vi "Write Ch.vi"(8 "error in":errorcluster, 9 "Channel":i32, 10 "Producer Ch":T1, 11 "Cycler Cluster - 24 Channel.lvclass":refnum<class "Cycler Cluster - 24 Channel.lvclass">) -> (0 "error out":errorcluster, 3 "output cluster":refnum<class "Cycler Cluster - 24 Channel.lvclass">)   [LabVIEW 2023, in "Cycler Cluster - 24 Channel.lvclass"]
uses:
  Cycler Cluster - 24 Channel.lvclass
  Cycler Cluster - 24 Channel.lvclass/Cycler Cluster - 24 Channel.ctl
  f4d7046b-01d5-476e-969f-edff788d7dd0.vi
  09ba8855-a333-4b05-9fa0-f00f0d112976.vi
  f692a3ce-3a89-48d1-896d-de4404ed547f.vi
  300b3033-2680-412c-ab22-c723e8d8dc08.vi
  7cf0eb00-689e-4e52-8b4d-642b65507f98.vi
  b87ff49e-8005-4a7c-bf49-406770351efc.vi
  dc6f3a3c-9a41-4b47-836c-8d10a2dd6bc9.vi
  5b0f37a0-0270-4c49-ba01-7464d39b0c09.vi
  d2784768-1ffd-4bb1-aa68-cb021ec6bd11.vi
  d58bec58-6c3c-4b44-9526-a74563a41a00.vi
  6f99bfdc-e3a0-47bf-9a28-a7b183ece507.vi
  03bc517d-3567-4243-82ce-a9681bd71644.vi
  cfb328b4-c11e-4fec-8c64-e5bccd80eed6.vi
  f724775c-be9e-4d2c-be3a-0a88198af531.vi
  bbda8b00-4939-44f4-9757-bc2aa60b7321.vi
  d38bd821-1f4e-4e4a-b7c3-0ef1bfe1a6e8.vi
  197e6fb9-9472-4794-b678-1f8964912596.vi
  48b47df3-7b2f-442d-868c-df429242df4d.vi
  13396400-6a8b-4566-8927-19bad4ed771a.vi
  f607f0d2-4827-4487-99bd-0b5c3bd37f17.vi
  8e66ad1f-a7de-4d63-a362-64d5987b21bd.vi
  6b9c6a2f-fe1c-43a7-87f9-81ce4a8c2619.vi
  de965fe8-e7e9-435a-96db-c6a4e30d0dc4.vi
  dd587189-f4e7-40a8-a0a0-060e1a74fe14.vi
  f4d7046b-01d5-476e-969f-edff788d7dd0.vi/4bc1c15b-36ab-481f-b8dd-c64075ce723a.vi
  f4d7046b-01d5-476e-969f-edff788d7dd0.vi/d83cb72b-7713-41fc-a3d1-682de79cf574.vi
  09ba8855-a333-4b05-9fa0-f00f0d112976.vi/4bc1c15b-36ab-481f-b8dd-c64075ce723a.vi
  09ba8855-a333-4b05-9fa0-f00f0d112976.vi/d83cb72b-7713-41fc-a3d1-682de79cf574.vi
  f692a3ce-3a89-48d1-896d-de4404ed547f.vi/4bc1c15b-36ab-481f-b8dd-c64075ce723a.vi
  f692a3ce-3a89-48d1-896d-de4404ed547f.vi/d83cb72b-7713-41fc-a3d1-682de79cf574.vi
  300b3033-2680-412c-ab22-c723e8d8dc08.vi/4bc1c15b-36ab-481f-b8dd-c64075ce723a.vi
  300b3033-2680-412c-ab22-c723e8d8dc08.vi/d83cb72b-7713-41fc-a3d1-682de79cf574.vi
  7cf0eb00-689e-4e52-8b4d-642b65507f98.vi/4bc1c15b-36ab-481f-b8dd-c64075ce723a.vi
  7cf0eb00-689e-4e52-8b4d-642b65507f98.vi/d83cb72b-7713-41fc-a3d1-682de79cf574.vi
  b87ff49e-8005-4a7c-bf49-406770351efc.vi/4bc1c15b-36ab-481f-b8dd-c64075ce723a.vi
  b87ff49e-8005-4a7c-bf49-406770351efc.vi/d83cb72b-7713-41fc-a3d1-682de79cf574.vi
  dc6f3a3c-9a41-4b47-836c-8d10a2dd6bc9.vi/4bc1c15b-36ab-481f-b8dd-c64075ce723a.vi
  dc6f3a3c-9a41-4b47-836c-8d10a2dd6bc9.vi/d83cb72b-7713-41fc-a3d1-682de79cf574.vi
  5b0f37a0-0270-4c49-ba01-7464d39b0c09.vi/4bc1c15b-36ab-481f-b8dd-c64075ce723a.vi
  5b0f37a0-0270-4c49-ba01-7464d39b0c09.vi/d83cb72b-7713-41fc-a3d1-682de79cf574.vi
  d2784768-1ffd-4bb1-aa68-cb021ec6bd11.vi/4bc1c15b-36ab-481f-b8dd-c64075ce723a.vi
  d2784768-1ffd-4bb1-aa68-cb021ec6bd11.vi/d83cb72b-7713-41fc-a3d1-682de79cf574.vi
  d58bec58-6c3c-4b44-9526-a74563a41a00.vi/4bc1c15b-36ab-481f-b8dd-c64075ce723a.vi
  d58bec58-6c3c-4b44-9526-a74563a41a00.vi/d83cb72b-7713-41fc-a3d1-682de79cf574.vi
  6f99bfdc-e3a0-47bf-9a28-a7b183ece507.vi/4bc1c15b-36ab-481f-b8dd-c64075ce723a.vi
  6f99bfdc-e3a0-47bf-9a28-a7b183ece507.vi/d83cb72b-7713-41fc-a3d1-682de79cf574.vi
  03bc517d-3567-4243-82ce-a9681bd71644.vi/4bc1c15b-36ab-481f-b8dd-c64075ce723a.vi
  03bc517d-3567-4243-82ce-a9681bd71644.vi/d83cb72b-7713-41fc-a3d1-682de79cf574.vi
  cfb328b4-c11e-4fec-8c64-e5bccd80eed6.vi/4bc1c15b-36ab-481f-b8dd-c64075ce723a.vi
  cfb328b4-c11e-4fec-8c64-e5bccd80eed6.vi/d83cb72b-7713-41fc-a3d1-682de79cf574.vi
  f724775c-be9e-4d2c-be3a-0a88198af531.vi/4bc1c15b-36ab-481f-b8dd-c64075ce723a.vi
  f724775c-be9e-4d2c-be3a-0a88198af531.vi/d83cb72b-7713-41fc-a3d1-682de79cf574.vi
  bbda8b00-4939-44f4-9757-bc2aa60b7321.vi/4bc1c15b-36ab-481f-b8dd-c64075ce723a.vi
  bbda8b00-4939-44f4-9757-bc2aa60b7321.vi/d83cb72b-7713-41fc-a3d1-682de79cf574.vi
  d38bd821-1f4e-4e4a-b7c3-0ef1bfe1a6e8.vi/4bc1c15b-36ab-481f-b8dd-c64075ce723a.vi
  d38bd821-1f4e-4e4a-b7c3-0ef1bfe1a6e8.vi/d83cb72b-7713-41fc-a3d1-682de79cf574.vi
  197e6fb9-9472-4794-b678-1f8964912596.vi/4bc1c15b-36ab-481f-b8dd-c64075ce723a.vi
  197e6fb9-9472-4794-b678-1f8964912596.vi/d83cb72b-7713-41fc-a3d1-682de79cf574.vi
  48b47df3-7b2f-442d-868c-df429242df4d.vi/4bc1c15b-36ab-481f-b8dd-c64075ce723a.vi
  48b47df3-7b2f-442d-868c-df429242df4d.vi/d83cb72b-7713-41fc-a3d1-682de79cf574.vi
  13396400-6a8b-4566-8927-19bad4ed771a.vi/4bc1c15b-36ab-481f-b8dd-c64075ce723a.vi
  13396400-6a8b-4566-8927-19bad4ed771a.vi/d83cb72b-7713-41fc-a3d1-682de79cf574.vi
  f607f0d2-4827-4487-99bd-0b5c3bd37f17.vi/4bc1c15b-36ab-481f-b8dd-c64075ce723a.vi
  f607f0d2-4827-4487-99bd-0b5c3bd37f17.vi/d83cb72b-7713-41fc-a3d1-682de79cf574.vi
  8e66ad1f-a7de-4d63-a362-64d5987b21bd.vi/4bc1c15b-36ab-481f-b8dd-c64075ce723a.vi
  8e66ad1f-a7de-4d63-a362-64d5987b21bd.vi/d83cb72b-7713-41fc-a3d1-682de79cf574.vi
  6b9c6a2f-fe1c-43a7-87f9-81ce4a8c2619.vi/4bc1c15b-36ab-481f-b8dd-c64075ce723a.vi
  6b9c6a2f-fe1c-43a7-87f9-81ce4a8c2619.vi/d83cb72b-7713-41fc-a3d1-682de79cf574.vi
  de965fe8-e7e9-435a-96db-c6a4e30d0dc4.vi/4bc1c15b-36ab-481f-b8dd-c64075ce723a.vi
  de965fe8-e7e9-435a-96db-c6a4e30d0dc4.vi/d83cb72b-7713-41fc-a3d1-682de79cf574.vi
  dd587189-f4e7-40a8-a0a0-060e1a74fe14.vi/4bc1c15b-36ab-481f-b8dd-c64075ce723a.vi
  dd587189-f4e7-40a8-a0a0-060e1a74fe14.vi/d83cb72b-7713-41fc-a3d1-682de79cf574.vi
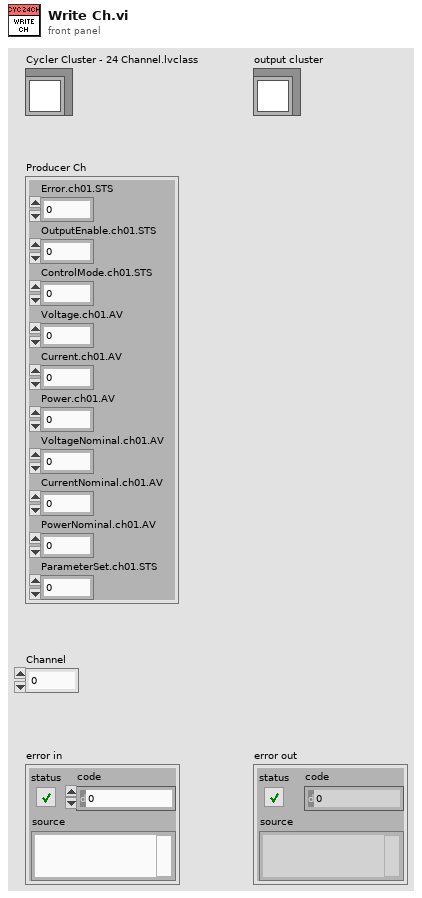
[diagram p1: front panel]
types:
  T1 = cluster{"Error.ch01.STS":i32, "OutputEnable.ch01.STS":i32, "ControlMode.ch01.STS":u16, "Voltage.ch01.AV":dbl, "Current.ch01.AV":dbl, "Power.ch01.AV":dbl, "VoltageNominal.ch01.AV":dbl, "CurrentNominal.ch01.AV":dbl, "PowerNominal.ch01.AV":dbl, "ParameterSet.ch01.STS":i32}
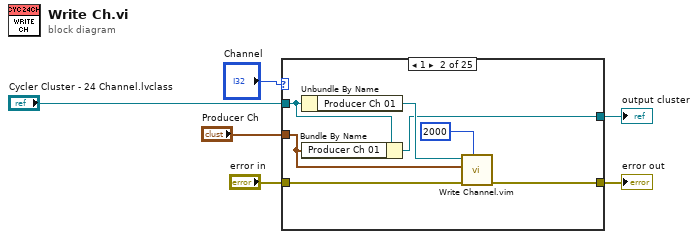
[diagram p0: block diagram]
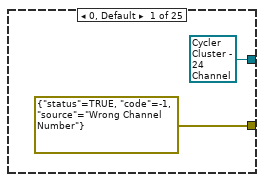
[diagram p2: hidden frame]
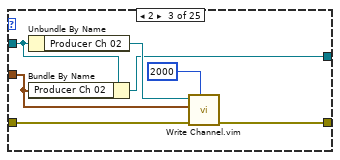
[diagram p3: hidden frame]
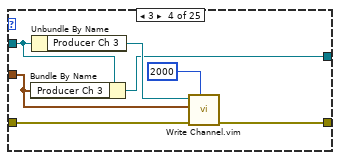
[diagram p4: hidden frame]
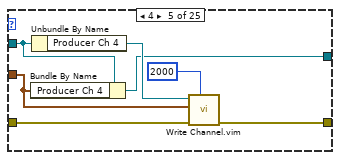
[diagram p5: hidden frame]
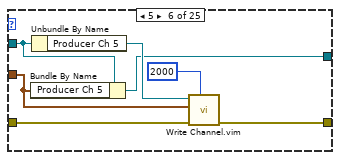
[diagram p6: hidden frame]
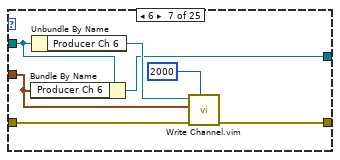
[diagram p7: hidden frame]
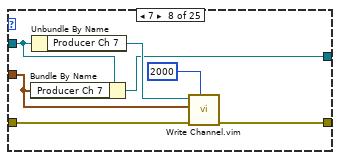
[diagram p8: hidden frame]
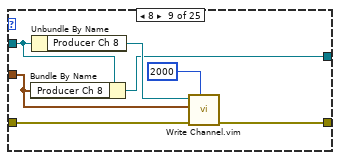
[diagram p9: hidden frame]
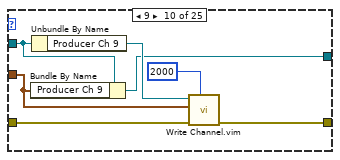
[diagram p10: hidden frame]
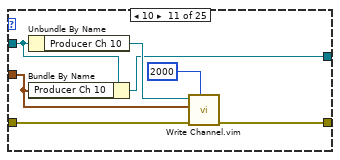
[diagram p11: hidden frame]
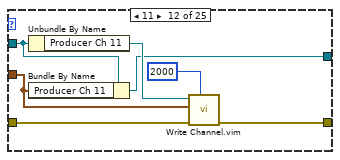
[diagram p12: hidden frame]
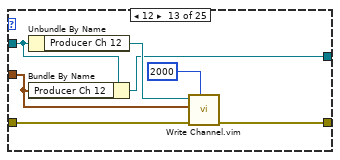
[diagram p13: hidden frame]
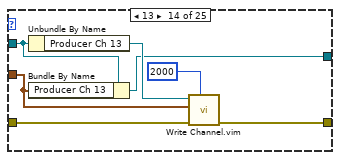
[diagram p14: hidden frame]
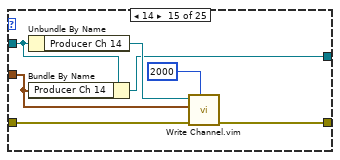
[diagram p15: hidden frame]
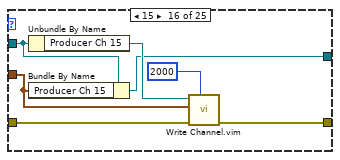
[diagram p16: hidden frame]
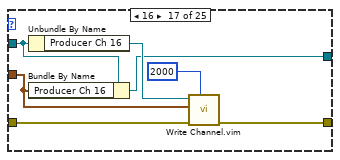
[diagram p17: hidden frame]
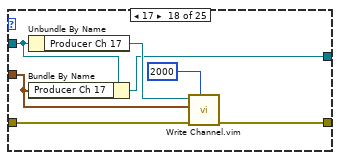
[diagram p18: hidden frame]
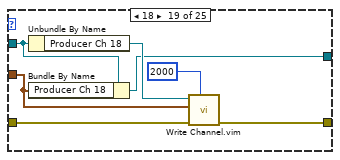
[diagram p19: hidden frame]
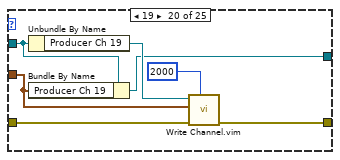
[diagram p20: hidden frame]
diagram:
  n1 = case shown="1" "Channel" {
    tunnel: "Producer Ch" -> [_ w12 w19 w26 w33 w40 w47 w54 w61 w68 w75 w82 w89 w96 w103 w110 w117 w124 w131 w138 w145 w152 w159 w166 w173]
    tunnel: "Cycler Cluster - 24 Channel.lvclass" -> [_ w13 w20 w27 w34 w41 w48 w55 w62 w69 w76 w83 w90 w97 w104 w111 w118 w125 w132 w139 w146 w153 w160 w167 w174]
    tunnel: [errorcluster {"status"=TRUE, "code"=-1, "source"="Wrong Channel Number"} ("error out") w11 w18 w25 w32 w39 w46 w53 w60 w67 w74 w81 w88 w95 w102 w109 w116 w123 w130 w137 w144 w151 w158 w165 w172] -> w3
    tunnel: "error in" -> [_ w10 w17 w24 w31 w38 w45 w52 w59 w66 w73 w80 w87 w94 w101 w108 w115 w122 w129 w136 w143 w150 w157 w164 w171]
    tunnel: [refnum<class "Cycler Cluster - 24 Channel.lvclass"> refnum ("Cycler Cluster - 24 Channel.lvclass") w9 w16 w23 w30 w37 w44 w51 w58 w65 w72 w79 w86 w93 w100 w107 w114 w121 w128 w135 w142 w149 w156 w163 w170] -> w1
    frame 0, Default {
    }
    frame 1 {
      n2 = Unbundle By Name(w13) -> ("Producer Ch 01"=w15:refnum<k21>)
      n3 = Bundle By Name(cluster=w13, "Producer Ch 01"=w12) -> (w9:refnum<class "Cycler Cluster - 24 Channel.lvclass">)
      n4 = call "Write Channel.vim"("Timeout (ms)"=2000, "error in"=w10, "Data in"=w12, "ADAS HIL Channel in"=w15) -> ("error out"=w11:errorcluster)  [unwired: 5 in, 2 out]
    }
    frame 2 {
      n5 = Unbundle By Name(w20) -> ("Producer Ch 02"=w22:refnum<k21>)
      n6 = Bundle By Name(cluster=w20, "Producer Ch 02"=w19) -> (w16:refnum<class "Cycler Cluster - 24 Channel.lvclass">)
      n7 = call "Write Channel.vim"("Timeout (ms)"=2000, "error in"=w17, "Data in"=w19, "ADAS HIL Channel in"=w22) -> ("error out"=w18:errorcluster)  [unwired: 5 in, 2 out]
    }
    frame 3 {
      n8 = Bundle By Name(cluster=w27, "Producer Ch 3"=w26) -> (w23:refnum<class "Cycler Cluster - 24 Channel.lvclass">)
      n9 = Unbundle By Name(w27) -> ("Producer Ch 3"=w29:refnum<k21>)
      n10 = call "Write Channel.vim"("Timeout (ms)"=2000, "error in"=w24, "Data in"=w26, "ADAS HIL Channel in"=w29) -> ("error out"=w25:errorcluster)  [unwired: 5 in, 2 out]
    }
    frame 4 {
      n11 = Bundle By Name(cluster=w34, "Producer Ch 4"=w33) -> (w30:refnum<class "Cycler Cluster - 24 Channel.lvclass">)
      n12 = Unbundle By Name(w34) -> ("Producer Ch 4"=w36:refnum<k21>)
      n13 = call "Write Channel.vim"("Timeout (ms)"=2000, "error in"=w31, "Data in"=w33, "ADAS HIL Channel in"=w36) -> ("error out"=w32:errorcluster)  [unwired: 5 in, 2 out]
    }
    frame 5 {
      n14 = Bundle By Name(cluster=w41, "Producer Ch 5"=w40) -> (w37:refnum<class "Cycler Cluster - 24 Channel.lvclass">)
      n15 = Unbundle By Name(w41) -> ("Producer Ch 5"=w43:refnum<k21>)
      n16 = call "Write Channel.vim"("Timeout (ms)"=2000, "error in"=w38, "Data in"=w40, "ADAS HIL Channel in"=w43) -> ("error out"=w39:errorcluster)  [unwired: 5 in, 2 out]
    }
    frame 6 {
      n17 = Bundle By Name(cluster=w48, "Producer Ch 6"=w47) -> (w44:refnum<class "Cycler Cluster - 24 Channel.lvclass">)
      n18 = Unbundle By Name(w48) -> ("Producer Ch 6"=w50:refnum<k21>)
      n19 = call "Write Channel.vim"("Timeout (ms)"=2000, "error in"=w45, "Data in"=w47, "ADAS HIL Channel in"=w50) -> ("error out"=w46:errorcluster)  [unwired: 5 in, 2 out]
    }
    frame 7 {
      n20 = Bundle By Name(cluster=w55, "Producer Ch 7"=w54) -> (w51:refnum<class "Cycler Cluster - 24 Channel.lvclass">)
      n21 = Unbundle By Name(w55) -> ("Producer Ch 7"=w57:refnum<k21>)
      n22 = call "Write Channel.vim"("Timeout (ms)"=2000, "error in"=w52, "Data in"=w54, "ADAS HIL Channel in"=w57) -> ("error out"=w53:errorcluster)  [unwired: 5 in, 2 out]
    }
    frame 8 {
      n23 = Bundle By Name(cluster=w62, "Producer Ch 8"=w61) -> (w58:refnum<class "Cycler Cluster - 24 Channel.lvclass">)
      n24 = Unbundle By Name(w62) -> ("Producer Ch 8"=w64:refnum<k21>)
      n25 = call "Write Channel.vim"("Timeout (ms)"=2000, "error in"=w59, "Data in"=w61, "ADAS HIL Channel in"=w64) -> ("error out"=w60:errorcluster)  [unwired: 5 in, 2 out]
    }
    frame 9 {
      n26 = Bundle By Name(cluster=w69, "Producer Ch 9"=w68) -> (w65:refnum<class "Cycler Cluster - 24 Channel.lvclass">)
      n27 = Unbundle By Name(w69) -> ("Producer Ch 9"=w71:refnum<k21>)
      n28 = call "Write Channel.vim"("Timeout (ms)"=2000, "error in"=w66, "Data in"=w68, "ADAS HIL Channel in"=w71) -> ("error out"=w67:errorcluster)  [unwired: 5 in, 2 out]
    }
    frame 10 {
      n29 = Unbundle By Name(w76) -> ("Producer Ch 10"=w78:refnum<k21>)
      n30 = Bundle By Name(cluster=w76, "Producer Ch 10"=w75) -> (w72:refnum<class "Cycler Cluster - 24 Channel.lvclass">)
      n31 = call "Write Channel.vim"("Timeout (ms)"=2000, "error in"=w73, "Data in"=w75, "ADAS HIL Channel in"=w78) -> ("error out"=w74:errorcluster)  [unwired: 5 in, 2 out]
    }
    frame 11 {
      n32 = Unbundle By Name(w83) -> ("Producer Ch 11"=w85:refnum<k21>)
      n33 = Bundle By Name(cluster=w83, "Producer Ch 11"=w82) -> (w79:refnum<class "Cycler Cluster - 24 Channel.lvclass">)
      n34 = call "Write Channel.vim"("Timeout (ms)"=2000, "error in"=w80, "Data in"=w82, "ADAS HIL Channel in"=w85) -> ("error out"=w81:errorcluster)  [unwired: 5 in, 2 out]
    }
    frame 12 {
      n35 = Unbundle By Name(w90) -> ("Producer Ch 12"=w92:refnum<k21>)
      n36 = Bundle By Name(cluster=w90, "Producer Ch 12"=w89) -> (w86:refnum<class "Cycler Cluster - 24 Channel.lvclass">)
      n37 = call "Write Channel.vim"("Timeout (ms)"=2000, "error in"=w87, "Data in"=w89, "ADAS HIL Channel in"=w92) -> ("error out"=w88:errorcluster)  [unwired: 5 in, 2 out]
    }
    frame 13 {
      n38 = Unbundle By Name(w97) -> ("Producer Ch 13"=w99:refnum<k21>)
      n39 = Bundle By Name(cluster=w97, "Producer Ch 13"=w96) -> (w93:refnum<class "Cycler Cluster - 24 Channel.lvclass">)
      n40 = call "Write Channel.vim"("Timeout (ms)"=2000, "error in"=w94, "Data in"=w96, "ADAS HIL Channel in"=w99) -> ("error out"=w95:errorcluster)  [unwired: 5 in, 2 out]
    }
    frame 14 {
      n41 = Unbundle By Name(w104) -> ("Producer Ch 14"=w106:refnum<k21>)
      n42 = Bundle By Name(cluster=w104, "Producer Ch 14"=w103) -> (w100:refnum<class "Cycler Cluster - 24 Channel.lvclass">)
      n43 = call "Write Channel.vim"("Timeout (ms)"=2000, "error in"=w101, "Data in"=w103, "ADAS HIL Channel in"=w106) -> ("error out"=w102:errorcluster)  [unwired: 5 in, 2 out]
    }
    frame 15 {
      n44 = Unbundle By Name(w111) -> ("Producer Ch 15"=w113:refnum<k21>)
      n45 = Bundle By Name(cluster=w111, "Producer Ch 15"=w110) -> (w107:refnum<class "Cycler Cluster - 24 Channel.lvclass">)
      n46 = call "Write Channel.vim"("Timeout (ms)"=2000, "error in"=w108, "Data in"=w110, "ADAS HIL Channel in"=w113) -> ("error out"=w109:errorcluster)  [unwired: 5 in, 2 out]
    }
    frame 16 {
      n47 = Unbundle By Name(w118) -> ("Producer Ch 16"=w120:refnum<k21>)
      n48 = Bundle By Name(cluster=w118, "Producer Ch 16"=w117) -> (w114:refnum<class "Cycler Cluster - 24 Channel.lvclass">)
      n49 = call "Write Channel.vim"("Timeout (ms)"=2000, "error in"=w115, "Data in"=w117, "ADAS HIL Channel in"=w120) -> ("error out"=w116:errorcluster)  [unwired: 5 in, 2 out]
    }
    frame 17 {
      n50 = Unbundle By Name(w125) -> ("Producer Ch 17"=w127:refnum<k21>)
      n51 = Bundle By Name(cluster=w125, "Producer Ch 17"=w124) -> (w121:refnum<class "Cycler Cluster - 24 Channel.lvclass">)
      n52 = call "Write Channel.vim"("Timeout (ms)"=2000, "error in"=w122, "Data in"=w124, "ADAS HIL Channel in"=w127) -> ("error out"=w123:errorcluster)  [unwired: 5 in, 2 out]
    }
    frame 18 {
      n53 = Unbundle By Name(w132) -> ("Producer Ch 18"=w134:refnum<k21>)
      n54 = Bundle By Name(cluster=w132, "Producer Ch 18"=w131) -> (w128:refnum<class "Cycler Cluster - 24 Channel.lvclass">)
      n55 = call "Write Channel.vim"("Timeout (ms)"=2000, "error in"=w129, "Data in"=w131, "ADAS HIL Channel in"=w134) -> ("error out"=w130:errorcluster)  [unwired: 5 in, 2 out]
    }
    frame 19 {
      n56 = Unbundle By Name(w139) -> ("Producer Ch 19"=w141:refnum<k21>)
      n57 = Bundle By Name(cluster=w139, "Producer Ch 19"=w138) -> (w135:refnum<class "Cycler Cluster - 24 Channel.lvclass">)
      n58 = call "Write Channel.vim"("Timeout (ms)"=2000, "error in"=w136, "Data in"=w138, "ADAS HIL Channel in"=w141) -> ("error out"=w137:errorcluster)  [unwired: 5 in, 2 out]
    }
    frame 20 {
      n59 = Unbundle By Name(w146) -> ("Producer Ch 20"=w148:refnum<k21>)
      n60 = Bundle By Name(cluster=w146, "Producer Ch 20"=w145) -> (w142:refnum<class "Cycler Cluster - 24 Channel.lvclass">)
      n61 = call "Write Channel.vim"("Timeout (ms)"=2000, "error in"=w143, "Data in"=w145, "ADAS HIL Channel in"=w148) -> ("error out"=w144:errorcluster)  [unwired: 5 in, 2 out]
    }
    frame 21 {
      n62 = Unbundle By Name(w153) -> ("Producer Ch 21"=w155:refnum<k21>)
      n63 = Bundle By Name(cluster=w153, "Producer Ch 21"=w152) -> (w149:refnum<class "Cycler Cluster - 24 Channel.lvclass">)
      n64 = call "Write Channel.vim"("Timeout (ms)"=2000, "error in"=w150, "Data in"=w152, "ADAS HIL Channel in"=w155) -> ("error out"=w151:errorcluster)  [unwired: 5 in, 2 out]
    }
    frame 22 {
      n65 = Unbundle By Name(w160) -> ("Producer Ch 22"=w162:refnum<k21>)
      n66 = Bundle By Name(cluster=w160, "Producer Ch 22"=w159) -> (w156:refnum<class "Cycler Cluster - 24 Channel.lvclass">)
      n67 = call "Write Channel.vim"("Timeout (ms)"=2000, "error in"=w157, "Data in"=w159, "ADAS HIL Channel in"=w162) -> ("error out"=w158:errorcluster)  [unwired: 5 in, 2 out]
    }
    frame 23 {
      n68 = Unbundle By Name(w167) -> ("Producer Ch 23"=w169:refnum<k21>)
      n69 = Bundle By Name(cluster=w167, "Producer Ch 23"=w166) -> (w163:refnum<class "Cycler Cluster - 24 Channel.lvclass">)
      n70 = call "Write Channel.vim"("Timeout (ms)"=2000, "error in"=w164, "Data in"=w166, "ADAS HIL Channel in"=w169) -> ("error out"=w165:errorcluster)  [unwired: 5 in, 2 out]
    }
    frame 24 {
      n71 = Unbundle By Name(w174) -> ("Producer Ch 24"=w176:refnum<k21>)
      n72 = Bundle By Name(cluster=w174, "Producer Ch 24"=w173) -> (w170:refnum<class "Cycler Cluster - 24 Channel.lvclass">)
      n73 = call "Write Channel.vim"("Timeout (ms)"=2000, "error in"=w171, "Data in"=w173, "ADAS HIL Channel in"=w176) -> ("error out"=w172:errorcluster)  [unwired: 5 in, 2 out]
    }
  }
  "error out" <- w3
  "output cluster" <- w1
